vi "Add Version Data to  ERD list.vi"(0 ".NET Refnum in":refnum<k24>, 1 "# of Iterations (Should be 2 except JL)":i32=2, 5 "GEA Inputs":T1={"Source"=229, "Destination"=192} {"Destination" format="%.0x"; "Source" format="%.0x"}, 9 "Read ERD List MC":T2[](array[typedef])=[{"ERD Number"=49, "Data Type"=enum."uint32_t"}, {"ERD Number"=127, "Data Type"=enum."string"}, {"ERD Number"=61467, "Data Type"=enum."uint8_t"}, {"ERD Number"=61457, "Data Type"=enum."string"}, {"ERD Number"=61459, "Data Type"=enum."string"}, {"ERD Number"=61460, "Data Type"=enum."string"}, {"ERD Number"=61461, "Data Type"=enum."uint16_t"}, {"ERD Number"=61462, "Data Type"=enum."uint16_t"}, {"ERD Number"=61468, "Data Type"=enum."string"}, {"ERD Number"=61483, "Data Type"=enum."string"}, {"ERD Number"=61582, "Data Type"=enum."string"}, {"ERD Number"=61478, "Data Type"=enum."string"}, {"ERD Number"=8275, "Data Type"=enum."string"}, {"ERD Number"=8272, "Data Type"=enum."string"}, {"ERD Number"=8269, "Data Type"=enum."string"}, {"ERD Number"=8262, "Data Type"=enum."string"}, {"ERD Number"=61495, "Data Type"=enum."string"}, {"ERD Number"=8266, "Data Type"=enum."string"}, {"ERD Number"=61501, "Data Type"=enum."string"}, {"ERD Number"=61510, "Data Type"=enum."string"}, {"ERD Number"=61594, "Data Type"=enum."string"}, {"ERD Number"=61597, "Data Type"=enum."string"}, {"ERD Number"=61443, "Data Type"=enum."string"}, {"ERD Number"=61503, "Data Type"=enum."string"}, {"ERD Number"=61619, "Data Type"=enum."string"}, {"ERD Number"=61618, "Data Type"=enum."string"}, {"ERD Number"=61611, "Data Type"=enum."string"}, {"ERD Number"=61613, "Data Type"=enum."string"}, {"ERD Number"=61615, "Data Type"=enum."string"}, {"ERD Number"=61605, "Data Type"=enum."string"}, {"ERD Number"=61626, "Data Type"=enum."string"}, {"ERD Number"=61624, "Data Type"=enum."string"}, {"ERD Number"=62242, "Data Type"=enum."string"}, {"ERD Number"=61463, "Data Type"=enum."string"}, {"ERD Number"=61608, "Data Type"=enum."string"}, {"ERD Number"=61609, "Data Type"=enum."string"}, {"ERD Number"=61719, "Data Type"=enum."string"}, {"ERD Number"=61555, "Data Type"=enum."string"}, {"ERD Number"=61567, "Data Type"=enum."string"}, {"ERD Number"=61568, "Data Type"=enum."string"}, {"ERD Number"=61549, "Data Type"=enum."string"}, {"ERD Number"=61610, "Data Type"=enum."string"}, {"ERD Number"=61600, "Data Type"=enum."string"}, {"ERD Number"=61677, "Data Type"=enum."string"}, {"ERD Number"=61554, "Data Type"=enum."string"}, {"ERD Number"=61565, "Data Type"=enum."string"}, {"ERD Number"=61566, "Data Type"=enum."string"}, {"ERD Number"=61743, "Data Type"=enum."string"}, {"ERD Number"=61744, "Data Type"=enum."string"}, {"ERD Number"=61556, "Data Type"=enum."string"}, {"ERD Number"=61557, "Data Type"=enum."string"}, {"ERD Number"=61479, "Data Type"=enum."string"}, {"ERD Number"=61698, "Data Type"=enum."string"}, {"ERD Number"=62214, "Data Type"=enum."string"}, {"ERD Number"=62215, "Data Type"=enum."string"}, {"ERD Number"=61607, "Data Type"=enum."string"}, {"ERD Number"=61563, "Data Type"=enum."string"}, {"ERD Number"=61628, "Data Type"=enum."string"}, {"ERD Number"=61617, "Data Type"=enum."string"}, {"ERD Number"=63510, "Data Type"=enum."string"}, {"ERD Number"=61728, "Data Type"=enum."string"}, {"ERD Number"=61729, "Data Type"=enum."string"}, {"ERD Number"=61736, "Data Type"=enum."string"}, {"ERD Number"=61737, "Data Type"=enum."string"}, {"ERD Number"=61738, "Data Type"=enum."string"}, {"ERD Number"=61739, "Data Type"=enum."string"}, {"ERD Number"=8193, "Data Type"=enum."string"}, {"ERD Number"=61606, "Data Type"=enum."string"}, {"ERD Number"=63489, "Data Type"=enum."string"}] {"ERD Number" format="%.0x"}, 11 "error in (no error)":errorcluster, 13 "#ERDs per message":i32=20) -> (4 "ERD Data Out out":T3[](array[typedef]) {"ERD Number" format="%.0x"}, 15 "error out":errorcluster)   [LabVIEW 2023]
uses:
  Common/LabVIEW GEA2 Toolkit/GEA3/type defs/ERD Read Data Out.ctl
  Common/LabVIEW GEA2 Toolkit/GEA3/type defs/ERD Read Data In.ctl
  Common/LabVIEW GEA2 Toolkit/GEA3/type defs/Source_Destination.ctl
  D:/Common/LabVIEW GEA2 Toolkit/source/GEA3 DLL Source/GeaCommunication.dll
  Common/LabVIEW GEA2 Toolkit/source/GEA3 DLL Source/GeaCommunication.dll
  Common/LabVIEW GEA2 Toolkit/GEA3/library/GEA2_Toolkit.lvlib
panel:
  out "Raw Data Out":string[](array[string])
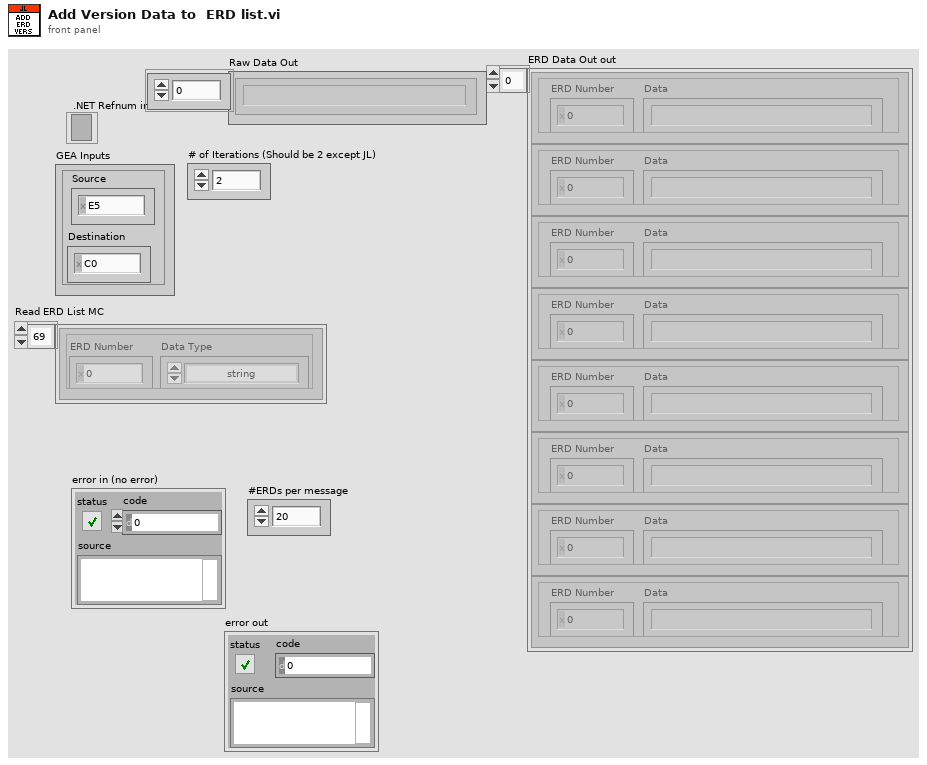
[diagram p1: front panel]
types:
  T1 = typedef "Source_Destination.ctl" = cluster{"Source":u8, "Destination":u8}
  T2 = typedef "ERD Read Data In.ctl" = cluster{"ERD Number":u16, "Data Type":enum16{"string", "boolean", "uint8_t", "uint16_t", "uint32_t", "uint64_t", "int8_t", "int16_t", "int32_t", "int64_t"}}
  T3 = typedef "ERD Read Data Out.ctl" = cluster{"ERD Number":u16, "Data":string}
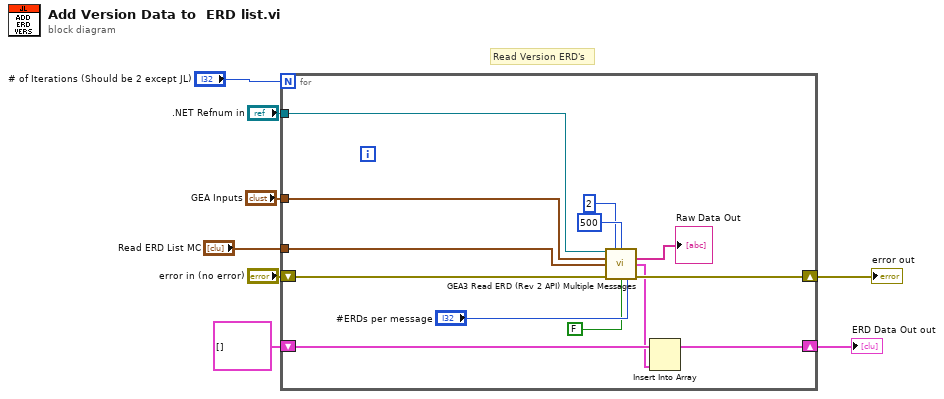
[diagram p0: block diagram]
diagram:
  # "Read Version ERD's"
  n1 = for {
    N: "# of Iterations (Should be 2 except JL)" -> [_]
    tunnel: ".NET Refnum in" -> [w18]
    tunnel: "GEA Inputs" -> [w14]
    tunnel: "Read ERD List MC" -> [w13]
    shift-right: [w19] -> w2
    shift-left: "error in (no error)" -> [w12]
    shift-right: [w15] -> w7
    shift-left: T3[] [] -> [w17]
    n2 = call "GEA3 Read ERD (Rev 2 API) Multiple Messages.vi"("GEA2 Reference In"=w18, "Retry Count"=2, "Read Timeout (ms)"=u32 500, "GEA Inputs"=w14, "Read ERD List"=w13, "Error In"=w12, "Verify ERD Response?"=FALSE, "Low Level Retry Count"="#ERDs per message") -> ("Raw Data Out"=→"Raw Data Out":string[], "ERD Data Out"=w16:cluster{"ERD Number":u16, "Data":string}[], "Error Out"=w19:errorcluster)  [unwired: 4 in, 1 out]
    n3 = Insert Into Array(array=w17, new element=w16) -> (w15:T3[])  [unwired: 1 in]
  }
  "ERD Data Out out" <- w7
  "error out" <- w2
